vi "USB3 Abort Get Buffer.vi"(8 "error in (no error)":errorcluster, 11 "hCamera":u32) -> (0 "error out":errorcluster, 2 "function return":i32, 3 "hCamera out":u32)   [LabVIEW 2013, in "Octoplus_LIDAR.lvlib"]
doc: "CAMCMOSOCTUSB3_API int __cdecl USB3_AbortGetBuffer(CAM_HANDLE hCamera);"
uses:
  <userlib>/Octoplus_LIDAR/Octoplus_LIDAR.lvlib
  <userlib>/Octoplus_LIDAR/CamCmosOctUsb3.dll
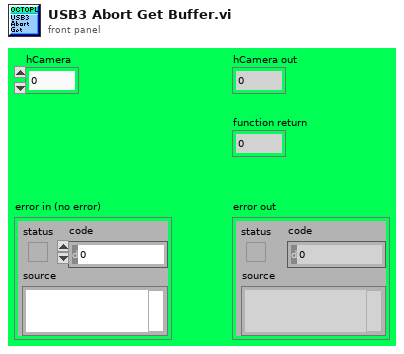
[diagram p1: front panel]
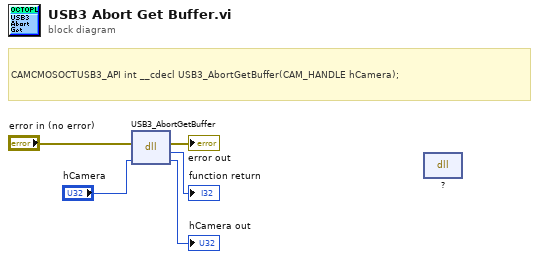
[diagram p0: block diagram]
diagram:
  # "CAMCMOSOCTUSB3_API int __cdecl USB3_AbortGetBuffer(CAM_HANDLE hCamera);"
  n1 = dll-call lib="C:/Program Files/National Instruments/LabVIEW 2013/user.lib/Octoplus_LIDAR/CamCmosOctUsb3.dll" fn="USB3_AbortGetBuffer"(error in="error in (no error)", "hCamera"="hCamera") -> (error out=→"error out":errorcluster, "return type"=→"function return":i32, "hCamera"=→"hCamera out":u32)  [unwired: 2 in, 1 out]
  n2 = dll-call lib="?" fn="?"() -> ()  [unwired: 4 in, 2 out]
